vi "Store Static VI References for Subpanel.vi"(8 "error in (no error)":errorcluster, 11 "HW with output config in":refnum<class "HW with output config.lvclass">) -> (0 "error out":errorcluster, 3 "HW with output config out":refnum<class "HW with output config.lvclass">)   [LabVIEW 2017, in "Hardware.lvlib" / "HW with output config.lvclass"]
uses:
  HW with output config.lvclass
  C:/Program Files (x86)/National Instruments/LabVIEW 2017/user.lib/Configuration Dialog Actor/Configuration.lvclass
  HW Config/Generation.vi
  HW Config/HW Configuration.lvclass
  <userlib>/Configuration Dialog Actor/Configuration.lvclass
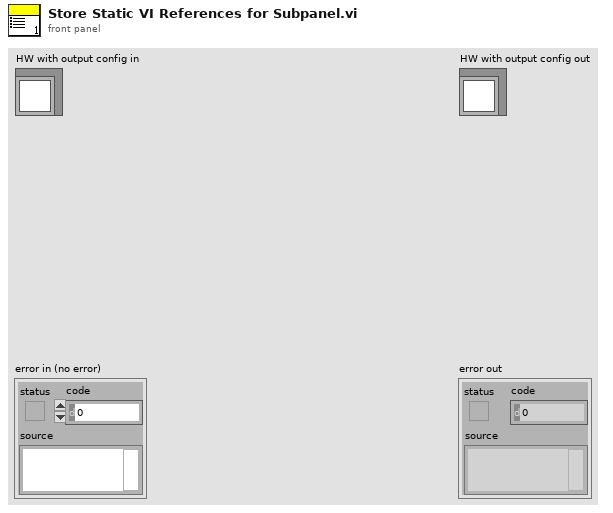
[diagram p1: front panel]
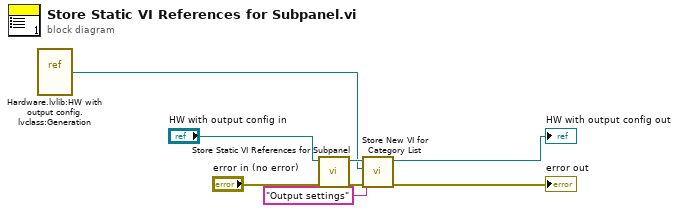
[diagram p0: block diagram]
diagram:
  n1 = vi-ref "Hardware.lvlib:HW with output config.lvclass:Generation.vi"() -> (w2:refnum<vi>)
  n2 = call-parent "Store Static VI References for Subpanel.vi"("error in (no error)"="error in (no error)", "HW Configuration in"="HW with output config in") -> ("error out"=w5:errorcluster, "HW Configuration out"=w6:refnum<class "HW with output config.lvclass">)  [unwired: 8 in]
  n3 = call <userlib>:"Store New VI for Category List.vi"("error in (no error)"=w5, "String"="Output settings", "VI Refnum"=w2, "Configuration in"=w6) -> ("error out"=→"error out":errorcluster, "Configuration out"=→"HW with output config out":refnum<class "HW with output config.lvclass">)  [unwired: 6 in]
